vi "Decider_BM_schwelle_dist_Huan.vi"(0 "Max. Wert Refl_1":dbl=0.00024, 1 "Abstand-Array-Refl 1":dbl=-144.07925033569336, 2 "stop abstand 1":dbl=50.0, 3 "Max. Wert Refl_2":dbl=0.0003214180438673588, 4 "Abstand-Array-Refl 2":dbl=77.92074966430664, 5 "stop abstand 2":dbl=80.0, 7 "Max. Wert Refl_3":dbl=0.00024, 9 "Abstand-Array-Refl 3":dbl=-144.07925033569336, 11 "stop abstand 3":dbl=35.0) -> (14 "R1-action":bool, 15 "R2-action":bool=TRUE, 16 "R3-action":bool, 17 "Prop 1":dbl=2.4000024000024e-10, 18 "Prop 2":dbl=4.124935209839127e-06, 19 "Prop 3":dbl=2.4000024000024e-10)   [LabVIEW 2014]
panel:
  out "R3 > 0,001":bool=TRUE
  out "R2 > 0,001":bool=TRUE
  out "R1 > 0,001":bool=TRUE
  out "d3<":bool
  out "R3>R2":bool
  out "R3>R1":bool
  out "d2<":bool=TRUE
  out "R2>R3":bool=TRUE
  out "R2>R1":bool=TRUE
  out "d1<":bool
  out "R1>R3":bool
  out "R1>R2":bool
  # "R2"
  # "R3"
  # "R1"
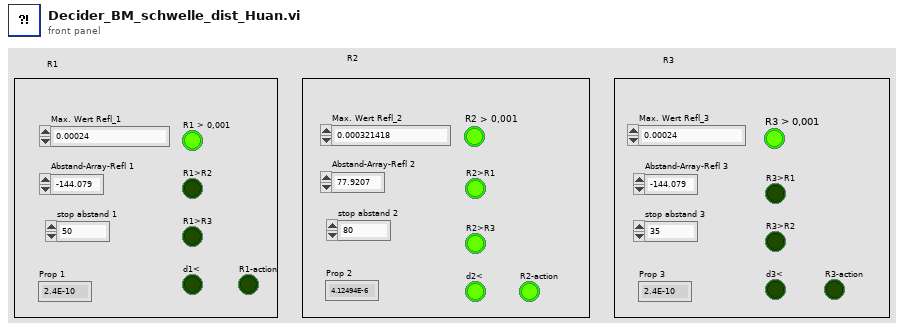
[diagram p1: front panel]
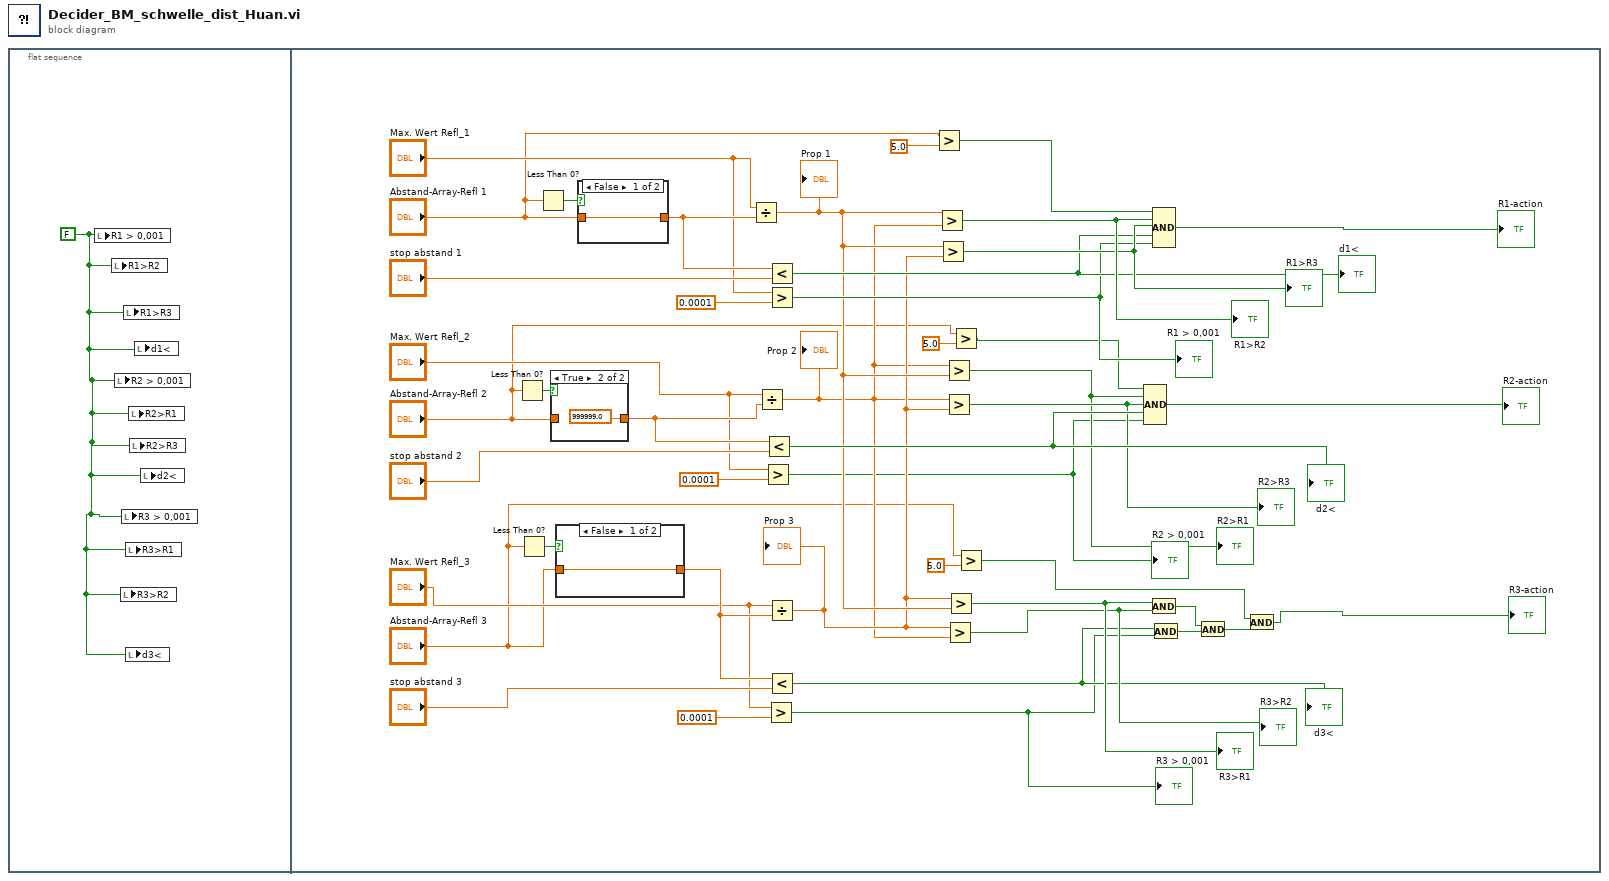
[diagram p0: block diagram]
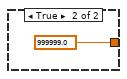
[diagram p2: hidden frame]
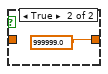
[diagram p4: hidden frame]
diagram:
  n1 = flat-sequence {
    frame #0 {
      w1 = FALSE
      n2 = local write "R1 > 0,001"(w1) -> ()
      n3 = local write "R1>R2"(w1) -> ()
      n4 = local write "R2 > 0,001"(w1) -> ()
      n5 = local write "R3>R2"(w1) -> ()
      n6 = local write "R3 > 0,001"(w1) -> ()
      n7 = local write "R1>R3"(w1) -> ()
      n8 = local write "R3>R1"(w1) -> ()
      n9 = local write "d3<"(w1) -> ()
      n10 = local write "R2>R1"(w1) -> ()
      n11 = local write "R2>R3"(w1) -> ()
      n12 = local write "d1<"(w1) -> ()
      n13 = local write "d2<"(w1) -> ()
    }
    frame #1 {
      n14 = Less Than 0?(x="Abstand-Array-Refl 2") -> (x < 0?=w45:bool)
      n15 = Less Than 0?(x="Abstand-Array-Refl 3") -> (x < 0?=w44:bool)
      n16 = Less Than 0?(x="Abstand-Array-Refl 1") -> (x < 0?=w46:bool)
      n17 = case shown="True" w45 {
        tunnel: "Abstand-Array-Refl 2" -> [w49 _]
        tunnel: [w49 999999.0 ("Abstand-Array-Refl 1")] -> w32
        frame False {
        }
        frame True {
        }
      }
      n18 = case shown="False" w44 {
        tunnel: "Abstand-Array-Refl 3" -> [w47 _]
        tunnel: [w47 999999.0 ("Abstand-Array-Refl 1")] -> w33
        frame False {
        }
        frame True {
        }
      }
      n19 = case shown="False" w46 {
        tunnel: "Abstand-Array-Refl 1" -> [w51 _]
        tunnel: [w51 999999.0 ("Abstand-Array-Refl 1")] -> w31
        frame False {
        }
        frame True {
        }
      }
      n20 = Divide(x="Max. Wert Refl_1", y=w31) -> (x/y=w22:dbl)
      "Prop 1" <- w22
      n21 = Divide(x="Max. Wert Refl_2", y=w32) -> (x/y=w20:dbl)
      "Prop 2" <- w20
      n22 = Greater?(x="Max. Wert Refl_2", y=0.0001) -> (0:w19:bool)
      "R2 > 0,001" <- w19
      n23 = Less?(x=w32, y="stop abstand 2") -> (x < y?=w40:bool)
      "d2<" <- w40
      n24 = Greater?(x="Max. Wert Refl_3", y=0.0001) -> (0:w7:bool)
      "R3 > 0,001" <- w7
      n25 = Less?(x=w31, y="stop abstand 1") -> (x < y?=w35:bool)
      "d1<" <- w35
      n26 = Greater?(x="Max. Wert Refl_1", y=0.0001) -> (0:w26:bool)
      "R1 > 0,001" <- w26
      n27 = Divide(x="Max. Wert Refl_3", y=w33) -> (x/y=w21:dbl)
      "Prop 3" <- w21
      n28 = Less?(x=w33, y="stop abstand 3") -> (x < y?=w8:bool)
      "d3<" <- w8
      n29 = Greater?(x="Abstand-Array-Refl 1", y=5.0) -> (0:w15:bool)
      n30 = Greater?(x=w22, y=w20) -> (0:w41:bool)
      "R1>R2" <- w41
      n31 = Greater?(x=w22, y=w21) -> (0:w39:bool)
      "R1>R3" <- w39
      n32 = Greater?(x=w20, y=w22) -> (0:w23:bool)
      "R2>R1" <- w23
      n33 = Greater?(x=w20, y=w21) -> (0:w38:bool)
      "R2>R3" <- w38
      n34 = Greater?(x=w21, y=w20) -> (0:w9:bool)
      "R3>R2" <- w9
      n35 = Greater?(x=w21, y=w22) -> (0:w10:bool)
      "R3>R1" <- w10
      n36 = Greater?(x="Abstand-Array-Refl 2", y=5.0) -> (0:w17:bool)
      n37 = Greater?(x="Abstand-Array-Refl 3", y=5.0) -> (0:w3:bool)
      n38 = Compound Arithmetic op=AND(w17, w23, w38, w40, w19) -> (→"R2-action":bool)
      n39 = And(x=w10, y=w9) -> (x .and. y?=w5:bool)
      n40 = And(x=w8, y=w7) -> (x .and. y?=w6:bool)
      n41 = Compound Arithmetic op=AND(w15, w41, w39, w35, w26) -> (→"R1-action":bool)
      n42 = And(x=w5, y=w6) -> (x .and. y?=w4:bool)
      n43 = And(x=w3, y=w4) -> (x .and. y?=→"R3-action":bool)
    }
  }
